vi "calculator.vi"() -> ()   [LabVIEW 2014]
uses:
  <vilib>/Utility/inputDevices.llb/keyboardAcquire.vi
  <vilib>/Utility/inputDevices.llb/closeKeyboard.vi
panel:
  in  "backspace":bool
  in  "9":bool
  in  "8":bool
  in  "4":bool
  in  "7":bool
  in  "3":bool
  in  "5":bool
  in  "2":bool
  in  "6":bool
  in  "1":bool
  in  "0":bool
  in  "off":bool
  in  "C":bool
  in  "equal":bool
  in  ".":bool
  in  "div":bool
  in  "sub":bool
  in  "mul":bool
  in  "add":bool
  out "showText":string
  # "1.2.1 --> 1.2"
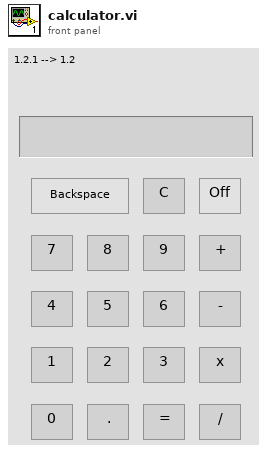
[diagram p1: front panel]
types:
  T1 = enum16{"0", "1", "2", "3", "4", "5", "6", "7", "8", "9", "A", "B", "C", "D", "E", "F", "G", "H", "I", "J", "K", "L", "M", "N", "O", "P", "Q", "R", "S", "T", "U", "V", "W", "X", "Y", "Z", "F1", "F2", "F3", "F4", "F5", "F6", "F7", "F8", "F9", "F10", "F11", "F12", "F13", "F14", "F15", "ADD", "BACK", "BACKSLASH", "CAPITAL", "COMMA", "DECIMAL", "DELETE", "DIVIDE", "DOWN", "END", "EQUALS", "ESCAPE", "GRAVE (`)", "HOME", "INSERT", "LBRACKET", "LCONTROL", "LEFT", "L ALT", "LSHIFT", "LWIN", "MINUS", "MULTIPLY", "NEXT", "NUMLOCK", "NUMPAD_0", "NUMPAD_1", "NUMPAD_2", "NUMPAD_3", "NUMPAD_4", "NUMPAD_5", "NUMPAD_6", "NUMPAD_7", "NUMPAD_8", "NUMPAD_9", "PAUSE", "PERIOD", "PRIOR (PG UP)", "RBRACKET", "RCONTROL", "RETURN", "RIGHT", "R ALT", "RSHIFT", "RWIN", "SCROLL", "SEMICOLON", "SLASH", "SPACE", "SUBTRACT", "TAB", "UP", "ENTER (num pad)", "' (quote)"}[]
  T2 = enum16{"0", "1", "2", "3", "4", "5", "6", "7", "8", "9", "A", "B", "C", "D", "E", "F", "G", "H", "I", "J", "K", "L", "M", "N", "O", "P", "Q", "R", "S", "T", "U", "V", "W", "X", "Y", "Z", "F1", "F2", "F3", "F4", "F5", "F6", "F7", "F8", "F9", "F10", "F11", "F12", "F13", "F14", "F15", "ADD", "BACK", "BACKSLASH", "CAPITAL", "COMMA", "DECIMAL", "DELETE", "DIVIDE", "DOWN", "END", "EQUALS", "ESCAPE", "GRAVE (`)", "HOME", "INSERT", "LBRACKET", "LCONTROL", "LEFT", "L ALT", "LSHIFT", "LWIN", "MINUS", "MULTIPLY", "NEXT", "NUMLOCK", "NUMPAD_0", "NUMPAD_1", "NUMPAD_2", "NUMPAD_3", "NUMPAD_4", "NUMPAD_5", "NUMPAD_6", "NUMPAD_7", "NUMPAD_8", "NUMPAD_9", "PAUSE", "PERIOD", "PRIOR (PG UP)", "RBRACKET", "RCONTROL", "RETURN", "RIGHT", "R ALT", "RSHIFT", "RWIN", "SCROLL", "SEMICOLON", "SLASH", "SPACE", "SUBTRACT", "TAB", "UP", "ENTER (num pad)", "' (quote)"}
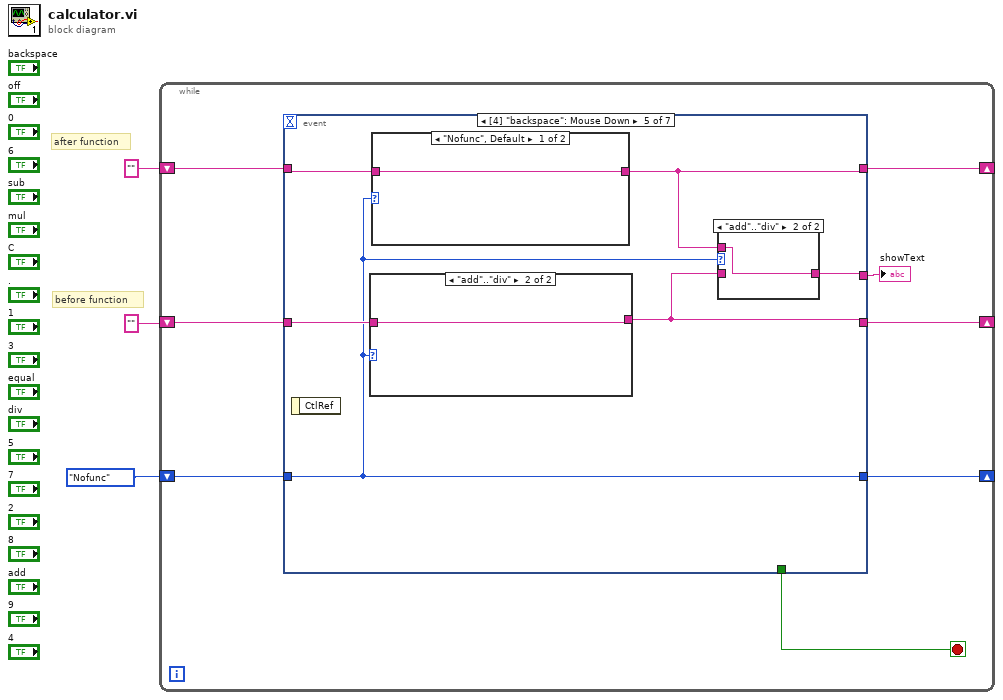
[diagram p0: block diagram]
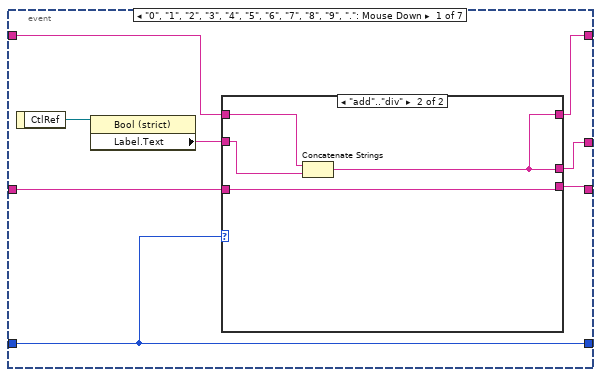
[diagram p2: hidden frame]
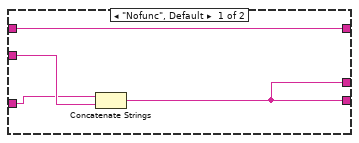
[diagram p3: hidden frame]
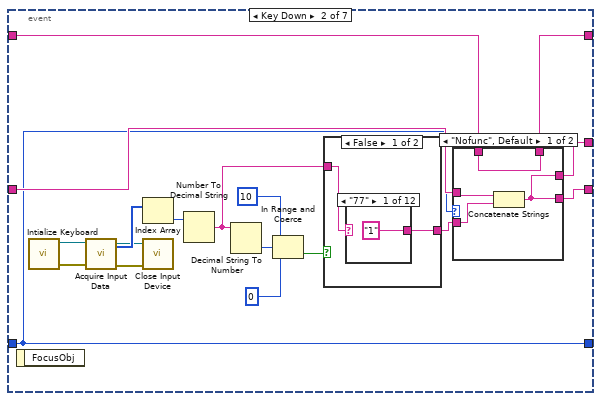
[diagram p4: hidden frame]
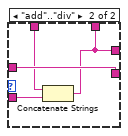
[diagram p5: hidden frame]
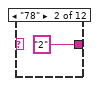
[diagram p6: hidden frame]
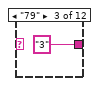
[diagram p7: hidden frame]
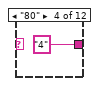
[diagram p8: hidden frame]
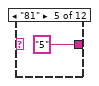
[diagram p9: hidden frame]
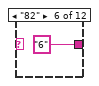
[diagram p10: hidden frame]
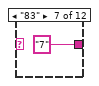
[diagram p11: hidden frame]
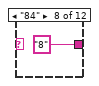
[diagram p12: hidden frame]
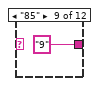
[diagram p13: hidden frame]
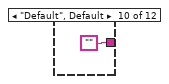
[diagram p14: hidden frame]
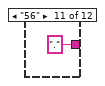
[diagram p15: hidden frame]
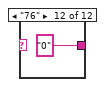
[diagram p16: hidden frame]
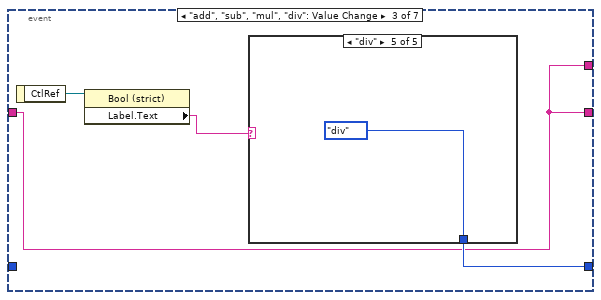
[diagram p18: hidden frame]
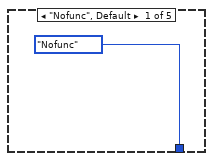
[diagram p19: hidden frame]
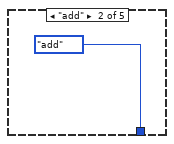
[diagram p20: hidden frame]
diagram:
  # "after function"
  # "before function"
  n1 = while {
    shift-right: [w11] -> _
    shift-left: "" -> [w8]
    shift-right: [w10] -> _
    shift-left: "" -> [w7]
    shift-right: [w9] -> _
    shift-left: enum16{"Nofunc", "add", "sub", "mul", "div"}."Nofunc" -> [w6]
    stop <- w4 stop-if-true
    n2 = event shown="[4] \"backspace\": Mouse Down" {
      selector: _ -> [_ _ _ _ _ _ _]
      dyn-events: _ -> [_ _ _ _ _ _ _]
      timeout: _ -> [_ _ _ _ _ _ _]
      tunnel: [w14 w29 _ w80 w119 w136 w138] -> w11
      tunnel: [w13 w31 w69 w79 w121 w136 w138] -> w10
      tunnel: [w16 w28 w70 _ w118 _ _] -> w9
      tunnel: w8 -> [w18 w30 _ w81 w122 _ _]
      tunnel: w7 -> [w17 w32 w69 w82 w123 _ _]
      tunnel: w6 -> [w16 w28 _ w83 w118 _ _]
      tunnel: [w12 w33 w69 w78 w120 w136 w138] -> w5
      tunnel: [_ _ _ _ _ _ TRUE] -> w4
      event "0", "1", "2", "3", "4", "5", "6", "7", "8", "9", ".": Mouse Down {
        n3 = event-data() -> ("CtlRef"=w19:refnum<vi>)  [unwired: 1 in]
        n4 = property class="Bool (strict)"(reference=w19) -> ("Label.Text"=w15:string)  [unwired: 1 in, 2 out]
        n5 = case shown="\"add\"..\"div\"" w16 {
          tunnel: w18 -> [w21 w26]
          tunnel: w17 -> [w22 w25]
          tunnel: w15 -> [w23 w27]
          tunnel: [w21 w24] -> w14
          tunnel: [w20 w25] -> w13
          tunnel: [w20 w24] -> w12
          frame "Nofunc", Default {
            n6 = Concatenate Strings(w22, w23) -> (w20:string)
          }
          frame "add".."div" {
            n7 = Concatenate Strings(w26, w27) -> (w24:string)
          }
        }
      }
      event Key Down {
        n8 = event-data() -> ()  [unwired: 1 in, 1 out]
        n9 = call <vilib>:"Intialize Keyboard.vi"() -> ("error out"=w39:errorcluster, "device ID"=w37:refnum<k1>)  [unwired: 10 in]
        n10 = call-poly <vilib>:"Acquire Input Data.vi"("device ID"=w37, "error in (no error)"=w39) -> ("device ID"=w38:refnum<k1>, "keys pressed"=w41:T1, "error out"=w40:errorcluster)  [unwired: 15 in]
        n11 = Index Array(array=w41) -> (element=w42:T2)  [unwired: 1 in]
        n12 = call-poly <vilib>:"Close Input Device.vi"("error in (no error)"=w40, "device ID"=w38) -> ()  [unwired: 8 in, 1 out]
        n13 = Number To Decimal String(number=w42) -> (decimal integer string=w44:string)  [unwired: 1 in]
        n14 = Decimal String To Number(string=w44) -> (number=w45:i32)  [unwired: 2 in, 1 out]
        n15 = In Range and Coerce(upper limit=10, x=w45, lower limit=0) -> (In Range?=w43:bool)  [unwired: 1 out]
        n16 = case shown="False" w43 {
          tunnel: [w55 w68] -> w34
          tunnel: w44 -> [w54 w68]
          frame False {
            n17 = case shown="\"77\"" w54 {
              tunnel: ["1" "2" "3" "4" "5" "6" "7" "8" "9" "" "." "0"] -> w55
              frame "77" {
              }
              frame "78" {
              }
              frame "79" {
              }
              frame "80" {
              }
              frame "81" {
              }
              frame "82" {
              }
              frame "83" {
              }
              frame "84" {
              }
              frame "85" {
              }
              frame "Default", Default {
              }
              frame "56" {
              }
              frame "76" {
              }
            }
          }
          frame True {
          }
        }
        n18 = case shown="\"Nofunc\", Default" w28 {
          tunnel: w34 -> [w49 w53]
          tunnel: [w47 w50] -> w33
          tunnel: [w46 w50] -> w29
          tunnel: w32 -> [w48 w52]
          tunnel: [w47 w52] -> w31
          tunnel: w30 -> [w46 w51]
          frame "Nofunc", Default {
            n19 = Concatenate Strings(w48, w49) -> (w47:string)
          }
          frame "add".."div" {
            n20 = Concatenate Strings(w51, w53) -> (w50:string)
          }
        }
      }
      event "add", "sub", "mul", "div": Value Change {
        n21 = event-data() -> ("CtlRef"=w72:refnum<vi>)  [unwired: 1 in]
        n22 = property class="Bool (strict)"(reference=w72) -> ("Label.Text"=w71:string)  [unwired: 1 in, 2 out]
        n23 = case shown="\"div\"" w71 {
          tunnel: [enum16{"Nofunc", "add", "sub", "mul", "div"}."Nofunc" enum16{"Nofunc", "add", "sub", "mul", "div"}."add" enum16{"Nofunc", "add", "sub", "mul", "div"}."sub" enum16{"Nofunc", "add", "sub", "mul", "div"}."mul" enum16{"Nofunc", "add", "sub", "mul", "div"}."div"] -> w70
          frame "Nofunc", Default {
          }
          frame "add" {
          }
          frame "sub" {
          }
          frame "mul" {
          }
          frame "div" {
          }
        }
      }
      event "equal": Mouse Down {
        n24 = event-data() -> ()  [unwired: 1 in, 1 out]
        n25 = case shown="\"sub\"" w83 {
          tunnel: [w85 "" "" "" ""] -> w80
          tunnel: [w84 "" "" "" ""] -> w79
          tunnel: [w85 w90 w100 w106 w114] -> w78
          tunnel: w82 -> [w84 w86 w96 w102 w113]
          tunnel: w81 -> [w85 w87 w97 w103 w112]
          frame "Nofunc", Default {
          }
          frame "add" {
            n26 = Fract/Exp String To Number(string=w87) -> (number=w91:dbl)  [unwired: 3 in, 1 out]
            n27 = Fract/Exp String To Number(string=w86) -> (number=w92:dbl)  [unwired: 3 in, 1 out]
            n28 = Add(x=w91, y=w92) -> (x+y=w93:dbl)
            n29 = Number To Fractional String(number=w93) -> (F-format string=w90:string)  [unwired: 3 in]
          }
          frame "sub" {
            n30 = Fract/Exp String To Number(string=w97) -> (number=w95:dbl)  [unwired: 3 in, 1 out]
            n31 = Fract/Exp String To Number(string=w96) -> (number=w94:dbl)  [unwired: 3 in, 1 out]
            n32 = Subtract(x=w94, y=w95) -> (x-y=w101:dbl)
            n33 = Number To Fractional String(number=w101) -> (F-format string=w100:string)  [unwired: 3 in]
          }
          frame "mul" {
            n34 = Fract/Exp String To Number(string=w103) -> (number=w107:dbl)  [unwired: 3 in, 1 out]
            n35 = Fract/Exp String To Number(string=w102) -> (number=w108:dbl)  [unwired: 3 in, 1 out]
            n36 = Multiply(x=w107, y=w108) -> (x*y=w109:dbl)
            n37 = Number To Fractional String(number=w109) -> (F-format string=w106:string)  [unwired: 3 in]
          }
          frame "div" {
            n38 = Fract/Exp String To Number(string=w112) -> (number=w110:dbl)  [unwired: 3 in, 1 out]
            n39 = Fract/Exp String To Number(string=w113) -> (number=w111:dbl)  [unwired: 3 in, 1 out]
            n40 = Divide(x=w111, y=w110) -> (x/y=w117:dbl)
            n41 = Number To Fractional String(number=w117) -> (F-format string=w114:string)  [unwired: 3 in]
          }
        }
      }
      event "backspace": Mouse Down {
        n42 = event-data() -> ()  [unwired: 1 in, 1 out]
        n43 = case shown="\"add\"..\"div\"" w118 {
          tunnel: w123 -> [w127 w130]
          tunnel: [w126 w130] -> w121
          frame "Nofunc", Default {
            n44 = String Length(string=w127) -> (length=w128:i32)
            n45 = Decrement(x=w128) -> (x-1=w129:i32)
            n46 = String Subset(string=w127, length (rest)=w129) -> (substring=w126:string)  [unwired: 1 in]
          }
          frame "add".."div" {
          }
        }
        n47 = case shown="\"Nofunc\", Default" w118 {
          tunnel: w122 -> [w131 w133]
          tunnel: [w131 w132] -> w119
          frame "Nofunc", Default {
          }
          frame "add".."div" {
            n48 = String Length(string=w133) -> (length=w135:i32)
            n49 = Decrement(x=w135) -> (x-1=w134:i32)
            n50 = String Subset(string=w133, length (rest)=w134) -> (substring=w132:string)  [unwired: 1 in]
          }
        }
        n51 = case shown="\"add\"..\"div\"" w118 {
          tunnel: w121 -> [w124 _]
          tunnel: [w124 w125] -> w120
          tunnel: w119 -> [_ w125]
          frame "Nofunc", Default {
          }
          frame "add".."div" {
          }
        }
      }
      event "C": Mouse Down {
        w136 = ""
        n52 = event-data() -> ()  [unwired: 1 in, 1 out]
      }
      event "off": Mouse Down {
        w138 = ""
        n53 = event-data() -> ()  [unwired: 1 in, 1 out]
      }
    }
    "showText" <- w5
  }
